vi "ExCloseGlobalCam.vi"() -> ()   [LabVIEW 2010]
uses:
  CamHandle.vi
panel:
  out "Camera open":bool
  out "error out":errorcluster
  in  "error in (no error)":errorcluster
  # "ExCloseGlobalCam: this subvi closes a camera that uses the gloabal\ncamera handle."
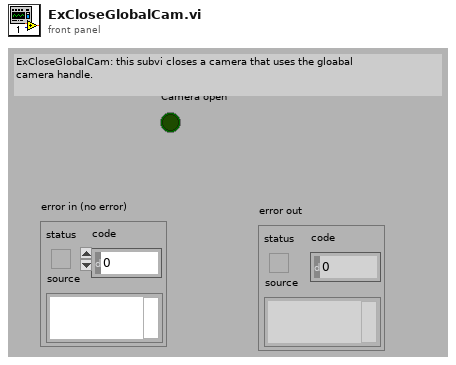
[diagram p1: front panel]
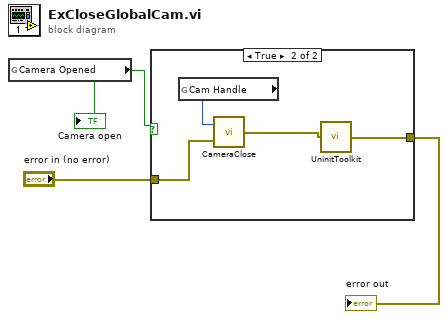
[diagram p0: block diagram]
diagram:
  n1 = global read "CamHandle.vi" "Camera Opened"() -> (w3:bool)
  "Camera open" <- w3
  n2 = case shown="True" w3 {
    tunnel: "error in (no error)" -> [w4 w8]
    tunnel: [w4 w6] -> w1
    frame False {
    }
    frame True {
      n3 = global read "CamHandle.vi" "Cam Handle"() -> (w5:u32)
      n4 = call <userlib>:"CameraClose.vi"("error in"=w8, "Camera Handle"=w5) -> ("error out"=w7:errorcluster)
      n5 = call <userlib>:"UninitToolkit.vi"("error in"=w7) -> ("error out"=w6:errorcluster)
    }
  }
  "error out" <- w1
